vi "Conversion_to_Volt.vi"(11 "Data":i16[](array[numeric])) -> (3 "Array":dbl[](array[numeric]))   [LabVIEW 2017]
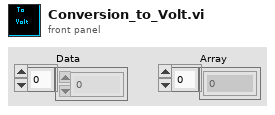
[diagram p1: front panel]
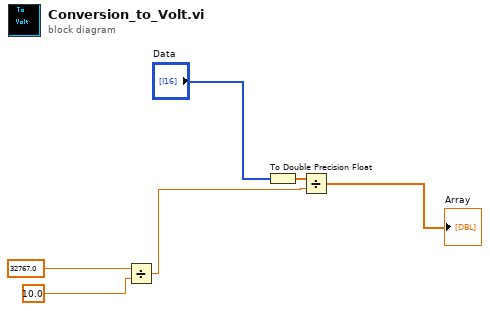
[diagram p0: block diagram]
diagram:
  n1 = Divide(x=32767.0, y=10.0) -> (x/y=w6:dbl)
  n2 = To Double Precision Float(number="Data") -> (double precision float=w1:dbl[])
  n3 = Divide(x=w1, y=w6) -> (x/y=→"Array":dbl[])
